vi "Register.vi"(8 "error in (no error)":errorcluster) -> (0 "error out":errorcluster)   [LabVIEW 2019, in "GaitDAQ UI.lvlib"]
uses:
  GaitDAQ UI.lvlib
panel:
  # "Input"
  # "Output"
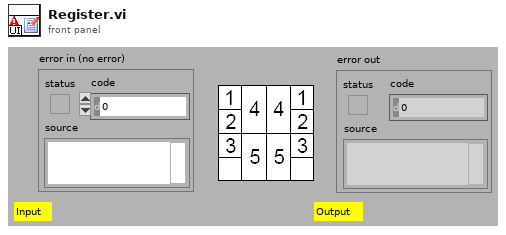
[diagram p1: front panel]
types:
  T1 = typedef "Event Message.lvlib/Event.ctl" = refnum<user-event>
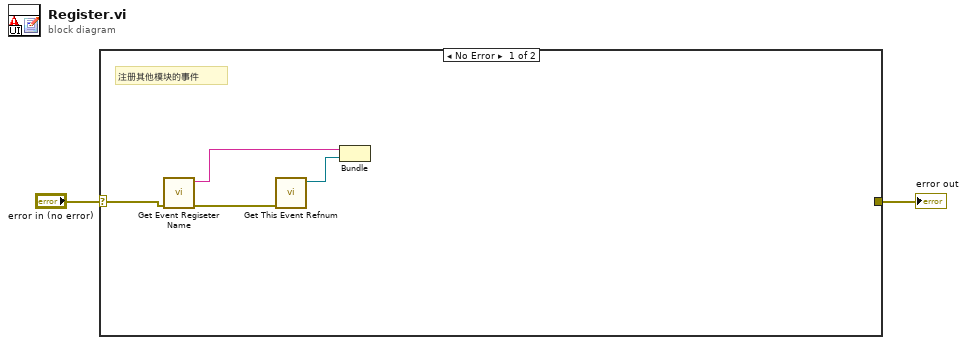
[diagram p0: block diagram]
diagram:
  n1 = case shown="No Error" "error in (no error)" {
    selector: "error in (no error)" -> [w3 w7]
    tunnel: [_ w7] -> w1
    frame No Error {
      # "注册其他模块的事件"
      n2 = call "Get Event Regiseter Name.vi"("error in (no error)"=w3) -> ("error out"=w4:errorcluster, "Event Register Name"=w5:string)  [unwired: 9 in]
      n3 = call "Get This Event Refnum.vi"("error in (no error)"=w4) -> ("This Event Refnum Out"=w6:T1)  [unwired: 9 in, 1 out]
      n4 = Bundle("Event Register Name"=w5, "This Event Refnum Out"=w6) -> ()  [unwired: 1 in, 1 out]
    }
    frame Error {
    }
  }
  "error out" <- w1
